vi "Define 2D Helmholtz PDE BC (VIRef).vi"(0 "PDE in":refnum<class "NI_PDE.lvclass">, 1 "data":variant, 5 "Boundary Condition":refnum<vi>, 7 "type":T2 items=["Dirichlet", "Neumann"], 9 "position":T1 items=["Start X", "End X", "Start Y", "End Y"], 11 "error in (no error)":errorcluster) -> (4 "PDE out":refnum<class "NI_PDE.lvclass">, 15 "error out":errorcluster)   [LabVIEW 2017, in "NI_PDE.lvlib"]
doc: "Defines the boundary condition of partial differential equations. You must manually select the polymorphic instance to use."
uses:
  <vilib>/gmath/NI_PDE.lvlib
  <vilib>/gmath/pde.llb/Common/PDE_BC Type.ctl
  <vilib>/gmath/pde.llb/PDEClass/NI_PDE.lvclass
  <vilib>/gmath/pde.llb/Common/PDE_BC Position 2D.ctl
  <vilib>/gmath/pde.llb/PDEClass/PDE_Helmholtz_2D/NI_PDE_Helmholtz_2D.lvclass
  e:/builds/penguin/labview/branches/2017/dev/dist/vi.lib/gmath/pde.llb/PDEClass/NI_PDE.lvclass
  <vilib>/gmath/pde.llb/BCClass/BC_Steady_2D_VIRef/NI_BC_Steady_2D_VIRef.lvclass
  e:/builds/penguin/labview/branches/2017/dev/dist/vi.lib/gmath/pde.llb/BCClass/NI_BC.lvclass
  <vilib>/gmath/pde.llb/BCClass/BC_Steady_2D_VIRef/BC Data.ctl
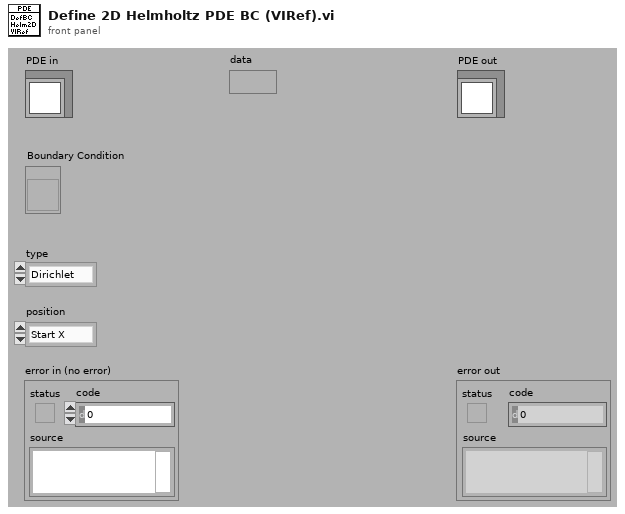
[diagram p1: front panel]
types:
  T1 = typedef "NI_PDE.lvlib/PDE_BC Position 2D.ctl" = i32
  T2 = typedef "NI_PDE.lvlib/PDE_BC Type.ctl" = i32
  T3 = typedef "NI_PDE.lvlib/NI_BC_Steady_2D_VIRef.lvclass/BC Data.ctl" = cluster{"type":T2, "position":T1, "G":refnum<vi>, "data":variant}
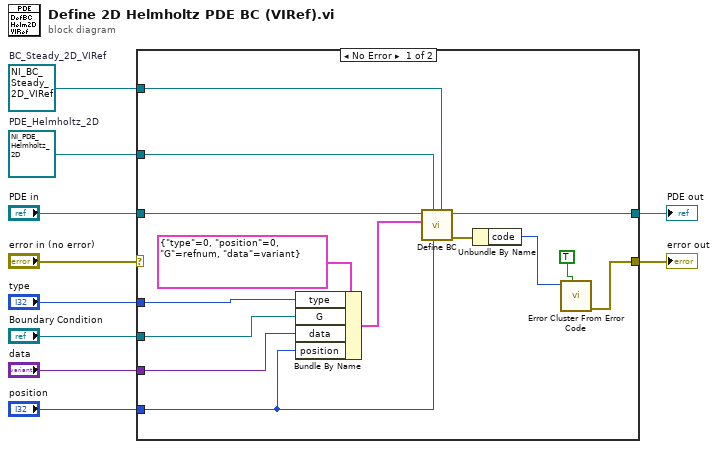
[diagram p0: block diagram]
diagram:
  w1 = refnum<class "NI_BC_Steady_2D_VIRef.lvclass"> refnum  # BC_Steady_2D_VIRef
  w3 = refnum<class "NI_PDE_Helmholtz_2D.lvclass"> refnum  # PDE_Helmholtz_2D
  n1 = case shown="No Error" "error in (no error)" {
    selector: "error in (no error)" -> [_ w25]
    tunnel: "PDE in" -> [w11 w26]
    tunnel: "position" -> [w15 _]
    tunnel: [w17 w26] -> w8
    tunnel: "Boundary Condition" -> [w19 _]
    tunnel: "type" -> [w20 _]
    tunnel: [w22 w25] -> w5
    tunnel: w3 -> [w14 _]
    tunnel: "data" -> [w18 _]
    tunnel: w1 -> [w13 _]
    frame No Error {
      n2 = Bundle By Name(cluster=T3 {"type"=0, "position"=0, "G"=refnum, "data"=variant} ("BC data"), "type"=w20, "G"=w19, "data"=w18, "position"=w15) -> (w12:T3)
      n3 = call <vilib>:"Define BC.vi"("target BC"=w13, "index"=w15, "target PDE"=w14, "BC"=w12, "PDE in"=w11) -> ("error out"=w16:errorcluster, "PDE out"=w17:refnum<class "NI_PDE.lvclass">)  [unwired: 2 in, 3 out]
      n4 = Unbundle By Name(w16) -> ("code"=w24:i32)
      n5 = call <vilib>:"Error Cluster From Error Code.vi"("show call chain? (False)"=TRUE, "error code (0)"=w24) -> ("error out"=w22:errorcluster)  [unwired: 1 in, 6 out]
    }
    frame Error {
    }
  }
  "PDE out" <- w8
  "error out" <- w5
